vi "GFITS_Parse_comment.vi"(10 "comment in":string, 11 "array in":string[][](table)) -> (2 "comment out":string, 3 "array out":string[][](table))   [LabVIEW 2016]
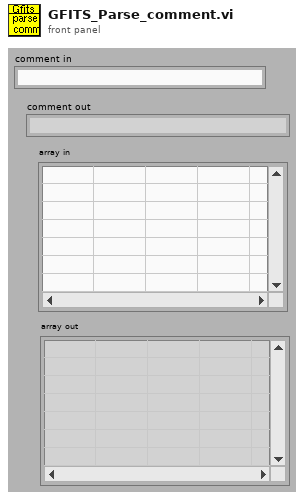
[diagram p1: front panel]
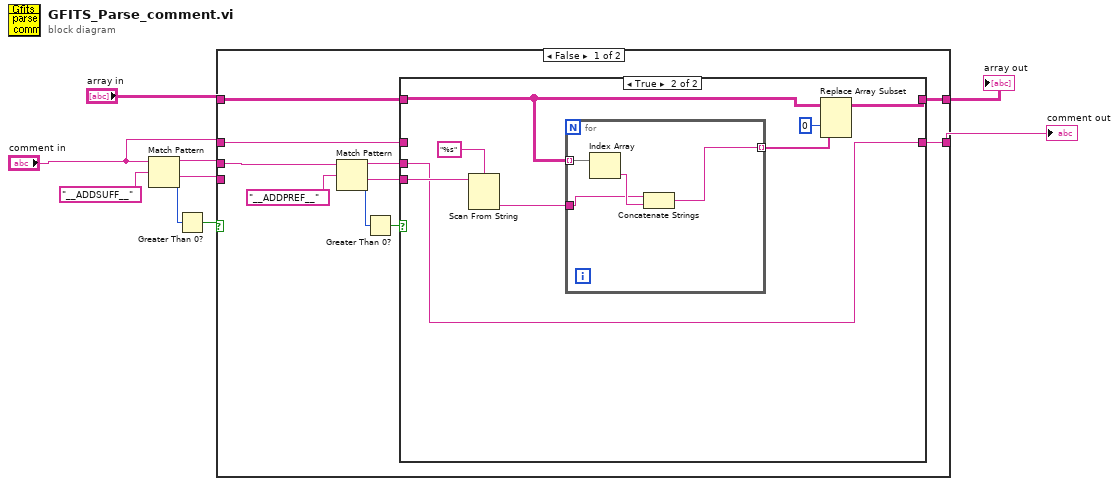
[diagram p0: block diagram]
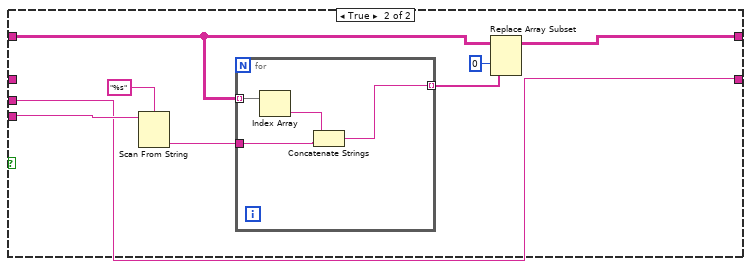
[diagram p3: hidden frame]
diagram:
  n1 = Match Pattern(string="comment in", regular expression="__ADDSUFF__") -> (before substring=w1:string, after substring=w6:string, offset past match=w8:i32)  [unwired: 2 out]
  n2 = Greater Than 0?(x=w8) -> (x > 0?=w7:bool)
  n3 = case shown="False" w7 {
    tunnel: w6 -> [_ w41]
    tunnel: "comment in" -> [w14 _]
    tunnel: [w13 w34] -> w4
    tunnel: "array in" -> [w16 w37]
    tunnel: [w12 w35] -> w2
    tunnel: w1 -> [w17 w34]
    frame False {
      n4 = Match Pattern(string=w17, regular expression="__ADDPREF__") -> (before substring=w10:string, after substring=w11:string, offset past match=w18:i32)  [unwired: 2 out]
      n5 = Greater Than 0?(x=w18) -> (x > 0?=w15:bool)
      n6 = case shown="True" w15 {
        tunnel: w16 -> [w20 w24]
        tunnel: w14 -> [w21 _]
        tunnel: [w21 w22] -> w13
        tunnel: [w20 w25] -> w12
        tunnel: w11 -> [_ w23]
        tunnel: w10 -> [_ w22]
        frame False {
        }
        frame True {
          n7 = Scan From String(format string="%s", input string=w23) -> (output 1=w28:string)  [unwired: 2 in, 4 out]
          n8 = for {
            tunnel: w28 -> [w30]
            tunnel: w24 -> [w33] mode=indexing
            tunnel: [w32] -> w26 mode=indexing
            n9 = Index Array(array=w33) -> (element=w31:string)  [unwired: 1 in]
            n10 = Concatenate Strings(w30, w31) -> (w32:string)
          }
          n11 = Replace Array Subset(array=w24, new element=w26, index (col)=0 ("disabled index (col)")) -> (w25:string[][])  [unwired: 1 in]
        }
      }
    }
    frame True {
      n12 = Scan From String(format string="%s", input string=w41) -> (output 1=w39:string)  [unwired: 2 in, 4 out]
      n13 = for {
        tunnel: w39 -> [w43]
        tunnel: w37 -> [w45] mode=indexing
        tunnel: [w42] -> w36 mode=indexing
        n14 = Index Array(array=w45) -> (element=w44:string)  [unwired: 1 in]
        n15 = Concatenate Strings(w44, w43) -> (w42:string)
      }
      n16 = Replace Array Subset(array=w37, new element=w36, index (col)=0 ("disabled index (col)")) -> (w35:string[][])  [unwired: 1 in]
    }
  }
  "comment out" <- w4
  "array out" <- w2
